vi "Initialize.vi"(8 "error in":errorcluster, 10 "shared resources":refnum<class "Shared Resources.lvclass">, 11 "Rx Execution Unit Implementation in":refnum<class "Rx Execution Unit.lvclass">) -> (0 "error out":errorcluster, 3 "Rx Execution Unit Implementation out":refnum<class "Rx Execution Unit.lvclass">)   [LabVIEW 2020, in "afdx_custom_device Engine.lvlib" / "Implementation.lvlib" / "Rx Execution Unit.lvclass"]
uses:
  Rx Execution Unit.lvclass
  Interfaces/Shared Resources/Shared Resources.lvclass
  Rx Execution Unit.lvclass/Rx Execution Unit.ctl
  AIM LabVIEW src/src/_polimorphicInstances/session/Fdx Create Session (RX-Monitor).vi
  AIM LabVIEW src/src/AIM664LV.lvlib
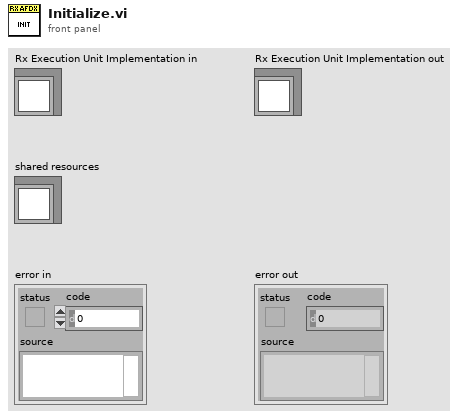
[diagram p1: front panel]
types:
  T1 = typedef "afdx_custom_device Engine.lvlib/Implementation.lvlib/Rx Execution Unit.lvclass/channel_settings_rx.ctl" = cluster{"Cluster":T2, "Rx Board":u32, "Rx Port":u32}
  T2 = typedef "AIM664LV.lvlib/session_monitor_config.ctl" = cluster{"DefaultCronoMode":u32, "GlbMonBufferSizeIn":u32}
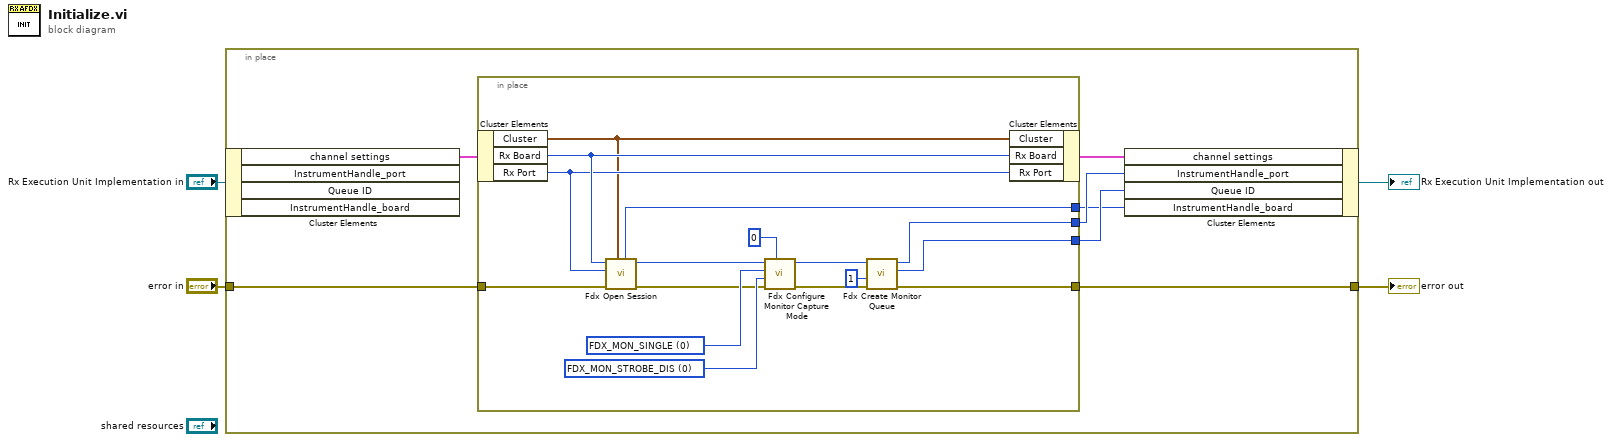
[diagram p0: block diagram]
diagram:
  n1 = in-place {
    in-place-border: "error in" -> [w10]
    in-place-border: [w6] -> w1
    n2 = in-place-cluster #1("Rx Execution Unit Implementation in") -> ("channel settings"=w11:T1)  [unwired: 3 out]
    n3 = in-place {
      in-place-border: w10 -> [w21]
      in-place-border: [w25] -> w8
      in-place-border: [w24] -> w7
      in-place-border: [w18] -> w6
      in-place-border: [w17] -> w5
      w16 = u32 0 items=["FDX_MON_STROBE_DIS", "FDX_MON_STROBE_STOP", "FDX_MON_STROBE_START"] ("Strobe")
      w15 = u32 0 items=["FDX_MON_SINGLE ", "FDX_MON_CONTINUOUS", "FDX_MON_SELECTIVE", "FDX_MON_RECORDING", "FDX_MON_REROS", "FDX_MON_HMU"] ("CaptureMode")
      n4 = in-place-cluster #2(w11) -> ("Cluster"=w19:T2, "Rx Board"=w23:u32, "Rx Port"=w22:u32)
      n5 = call-poly "Fdx Open Session.vi"("MonitorConfig"=w19, "error in (no error)"=w21, "port"=w22, "board"=w23) -> ("error out"=w12:errorcluster, "InstrumentHandle_port out"=w27:u32, "InstrumentHandle_board out"=w17:u32)  [unwired: 2 in, 3 out]
      n6 = call "Fdx Configure Monitor Capture Mode.vi"("TriggerPosition"=u32 0, "error in"=w12, "Strobe"=w16, "CaptureMode"=w15, "InstrumentHandle_port in"=w27) -> ("error out"=w20:errorcluster, "InstrumentHandle_port out"=w26:u32)  [unwired: 5 in]
      n7 = call "Fdx Create Monitor Queue.vi"("error in (no error)"=w20, "MaxFileSize MB (1)"=u32 1, "InstrumentHandle_port in"=w26) -> ("error out"=w18:errorcluster, "QueueIdOut"=w25:u32, "InstrumentHandle_port out"=w24:u32)  [unwired: 5 in, 1 out]
      n8 = in-place-cluster #2("Cluster"=w19, "Rx Board"=w23, "Rx Port"=w22) -> (w9:T1)
    }
    n9 = in-place-cluster #1("channel settings"=w9, "InstrumentHandle_port"=w7, "Queue ID"=w8, "InstrumentHandle_board"=w5) -> (→"Rx Execution Unit Implementation out":refnum<class "Rx Execution Unit.lvclass">)
  }
  "error out" <- w1
